vi "Open WebSocket.vi"(8 "error in (no error)":errorcluster, 11 "OBS in":refnum<class "OBS.lvclass">) -> (0 "error out":errorcluster, 3 "OBS out":refnum<class "OBS.lvclass">)   [LabVIEW 2022 SP3, in "obs-websocket-lv.lvlib" / "OBS.lvclass"]
uses:
  OBS.lvclass
  OBS.lvclass/OBS.ctl
  <vilib>/MediaMongrels Ltd/WebSockets/WebSockets/WebSocket Client/WebSocket Client.lvclass
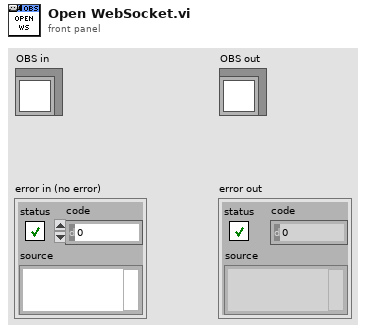
[diagram p1: front panel]
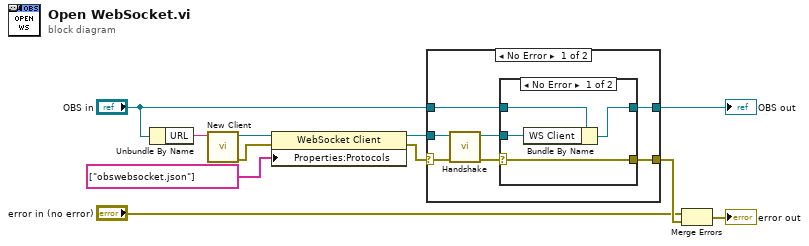
[diagram p0: block diagram]
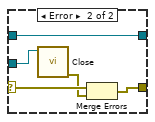
[diagram p2: hidden frame]
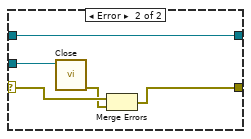
[diagram p3: hidden frame]
diagram:
  n1 = Unbundle By Name("OBS in") -> ("URL"=w11:string)
  n2 = call <vilib>:"New Client.vi"("WebSocket URL"=w11) -> ("error out"=w7:errorcluster, "WebSocket Client out"=w9:refnum<class "WebSocket Client.lvclass">)  [unwired: 9 in]
  n3 = property class="WebSocket Client"(reference=w9, error in=w7, "Properties:Protocols"=string[] ["obswebsocket.json"] ("Protocols")) -> (reference out=w6:refnum<class "WebSocket Client.lvclass">, error out=w5:errorcluster)
  n4 = case shown="No Error" w5 {
    selector: w5 -> [w16 w31]
    tunnel: "OBS in" -> [w18 w32]
    tunnel: [w12 w32] -> w1
    tunnel: w6 -> [w17 w28]
    tunnel: [w13 w30] -> w10
    frame No Error {
      n5 = call-dynamic "Handshake.vi"("error in (no error)"=w16, "WebSocket Client in"=w17) -> ("error out"=w14:errorcluster, "WebSocket Client out"=w15:refnum<class "WebSocket Client.lvclass">)  [unwired: 8 in]
      n6 = case shown="No Error" w14 {
        selector: w14 -> [w20 w25]
        tunnel: w18 -> [w22 w27]
        tunnel: [w20 w23] -> w13
        tunnel: [w19 w27] -> w12
        tunnel: w15 -> [w21 w26]
        frame No Error {
          n7 = Bundle By Name(cluster=w22, "WS Client"=w21) -> (w19:refnum<class "OBS.lvclass">)
        }
        frame Error {
          n8 = call-dynamic "Close.vi"("WebSocket in"=w26) -> ("error out"=w24:errorcluster)  [unwired: 10 in]
          n9 = Merge Errors(w25, w24) -> (w23:errorcluster)
        }
      }
    }
    frame Error {
      n10 = call-dynamic "Close.vi"("WebSocket in"=w28) -> ("error out"=w29:errorcluster)  [unwired: 10 in]
      n11 = Merge Errors(w31, w29) -> (w30:errorcluster)
    }
  }
  "OBS out" <- w1
  n12 = Merge Errors("error in (no error)", w10) -> (→"error out":errorcluster)
